vi "executeCommand.vi"(8 "error in (no error)":errorcluster, 9 "Variant":variant, 10 "commands":T1, 11 "DomeController in":refnum<class "DomeController.lvclass">) -> (0 "error out":errorcluster, 3 "DomeController out":refnum<class "DomeController.lvclass">)   [LabVIEW 2016, in "DomeController.lvclass"]
uses:
  DomeController.lvclass
  domeCommunicator/ComTypedefs/commands.ctl
  DomeController.lvclass/DomeController.ctl
  domeCommunicator/DomeCommunicator.lvclass
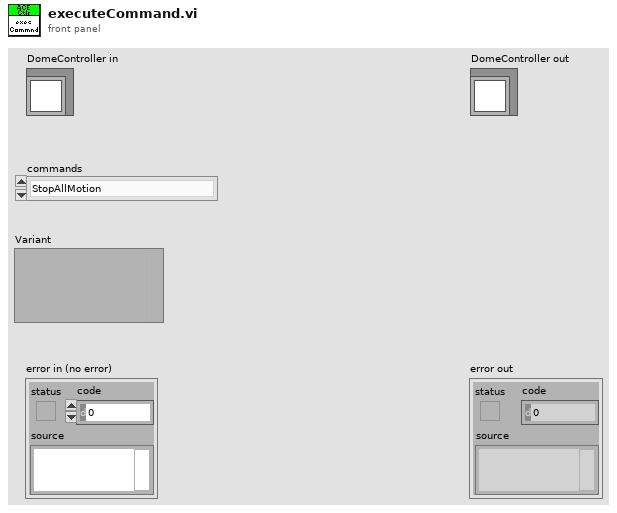
[diagram p1: front panel]
types:
  T1 = typedef "commands.ctl" = enum16{"StopAllMotion", "CloseMainDoor", "OpenMainDoor", "CloseDropoutDoor", "OpenDropoutDoor", "SynchronizedOpen", "SynchronizedClose", "AutoShutDownOn", "AutoShutDownOff", "RainOn", "RainOff", "CloudSensorOn", "CloudSensorOff", "RotateToHomePosition", "MoveToAzimuth", "SetTolerance", "DefineHomePosition", "HighSpeedThreshold", "SetCoast", "SetEncoderCountFor360", "SetWatchDogTimer", "SetReverseDirectionMotionDelay", "SaveCurrentConfiguration"}
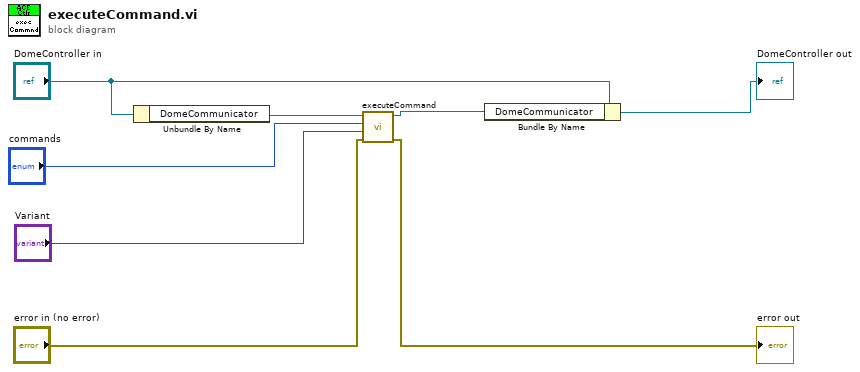
[diagram p0: block diagram]
diagram:
  n1 = Unbundle By Name("DomeController in") -> ("DomeCommunicator"=w7:refnum<class "DomeCommunicator.lvclass">)
  n2 = call "executeCommand.vi"("error in (no error)"="error in (no error)", "Variant"="Variant", "Command"="commands", "DomeCommunicator in"=w7) -> ("error out"=→"error out":errorcluster, "DomeCommunicator out"=w6:refnum<class "DomeCommunicator.lvclass">)  [unwired: 6 in]
  n3 = Bundle By Name(cluster="DomeController in", "DomeCommunicator"=w6) -> (→"DomeController out":refnum<class "DomeController.lvclass">)
